vi "WritePointToMem.vi"(10 "Point":cluster{"X":i32, "Y":i32, "Z":i32}, 11 "PointNum":u32) -> ()   [LabVIEW 2014]
uses:
  <vilib>/Platform/TimedLoop/XDataNode/timing_clust.ctl
  <vilib>/Platform/TimedLoop/XDataNode/nitl_modes.ctl
  <vilib>/Platform/TimedLoop/XDataNode/wakeup.ctl
  <vilib>/rvi/Emulation/niFpgaSctlEmulationGetInTimedLoop.vi
  <vilib>/rvi/Emulation/niFpgaEmulationReportErrorSimple.vi
  <vilib>/rvi/Emulation/niFpgaGetClockAttributes.vi
  <vilib>/rvi/Emulation/niFpgaCriticalErrorInLSC.vi
  <vilib>/rvi/eio/common/nirviEmuTemplateMethod_errors.vi
  <vilib>/Platform/TimedLoop/XDataNode/XDataNode.xnode
  <vilib>/eio/EIONode/EIONode.xnode
  <vilib>/Platform/TimedLoop/XDataNode/XDNodeRunTimeDep.lvlib
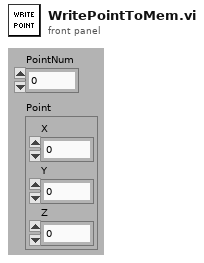
[diagram p1: front panel]
types:
  T1 = typedef "XDNodeRunTimeDep.lvlib/timing_clust.ctl" = cluster{"Expected End [f-1]":u64, "Actual End [f-1]":u64, "Finished Late? [f-1]":bool, "Expected End [i-1]":u64, "Actual End [i-1]":u64, "Finished Late? [i-1]":bool, "Expected Start [i]":u64, "Actual Start [i]":u64, "Expected Start [f]":u64, "Actual Start [f]":u64, "Source Name":string, "Structure Name":string, "Period":i64, "Deadline":i64, "Offset":i64, "Start":i64, "Priority":i32, "Timeout":i32, "Mode":T2, "Wakeup Reason":T3, "Error":errorcluster, "Source Type":string, "Secondary Source Type":string, "Global End Time":u64, "Global Start Time":u64, "Frame Duration":u64, "Iteration Duration":u64, "Assigned CPU":i32, "I/O Scan Engine Mode":u32}
  T2 = typedef "XDNodeRunTimeDep.lvlib/nitl_modes.ctl" = enum32{"No Change", "Process missed periods, maintain original phase", "Discard missed periods, maintain original phase", "Process missed periods, ignore original phase", "Discard missed periods, ignore original phase"}
  T3 = typedef "XDNodeRunTimeDep.lvlib/wakeup.ctl" = enum32{"Normal", "Aborted", "Asynchronous wakeup", "Timing source error", "Timed loop error", "Timeout"}
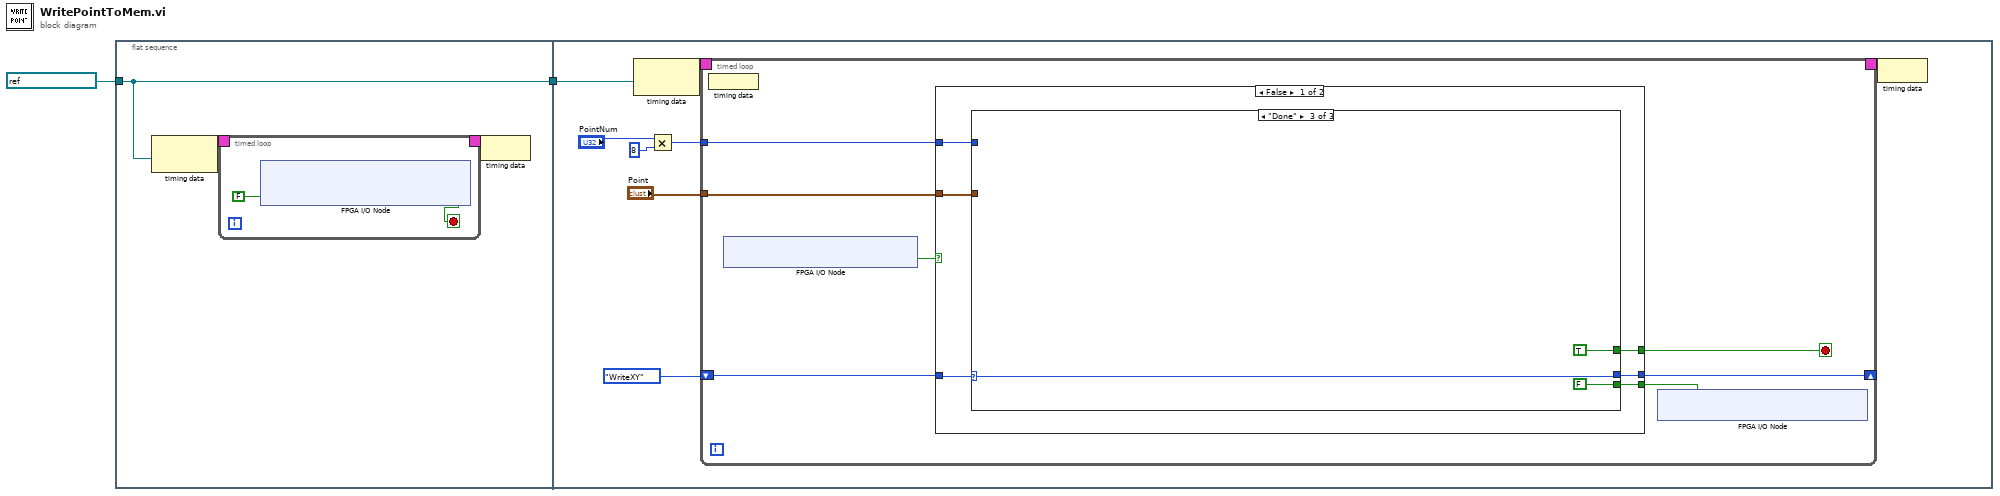
[diagram p0: block diagram]
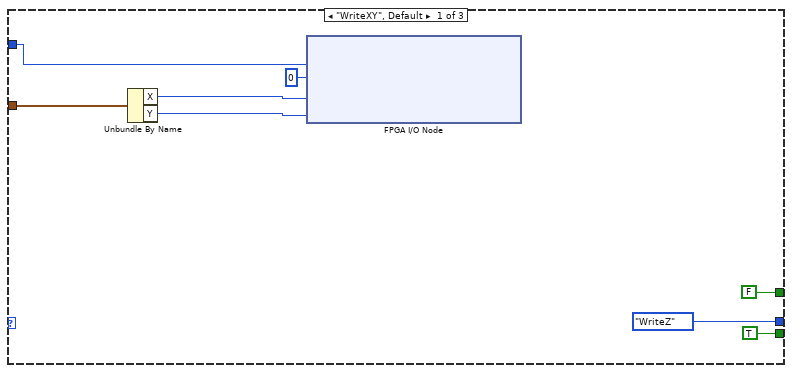
[diagram p2: hidden frame]
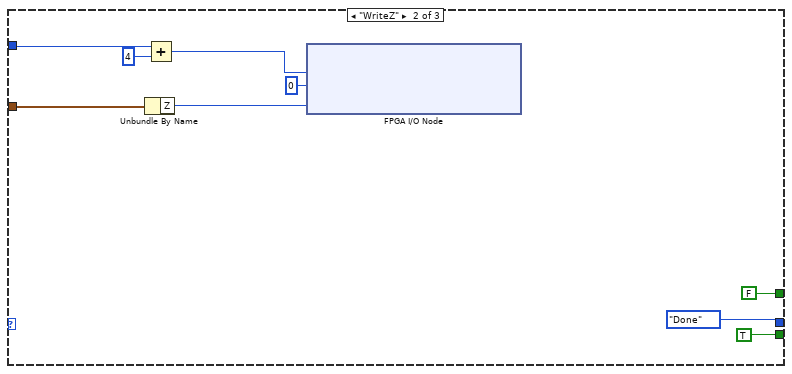
[diagram p3: hidden frame]
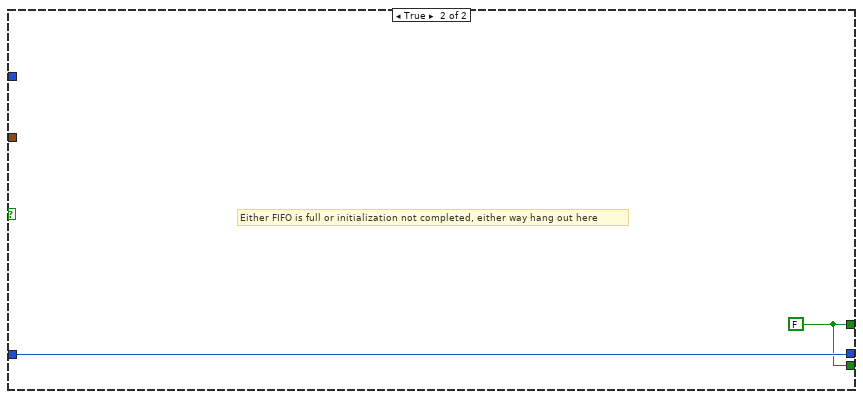
[diagram p4: hidden frame]
diagram:
  n1 = flat-sequence {
    tunnel: refnum<k21> "100 MHz Clock" ("Source Name") -> [w3]
    tunnel: [w3] -> w1
    tunnel: w1 -> [w14]
    frame #0 {
      n2 = node-c288(w3) -> (w5:T1)
      n3 = timed-loop {
        timing: w5 -> [_]
        timing-out: [_] -> w4
        stop <- w7 stop-if-true
        n4 = xnode "FPGA I/O Node"("DRAM Bank 0\\Command_Write_Enable"=FALSE ("DRAM Bank 0\\Command_Write_Enable")) -> ("DRAM Bank 0\\Initialization_Done"=w7:bool)  [unwired: 2 in, 2 out]
      }
      n5 = node-c288(w4) -> ()
    }
    frame #1 {
      n6 = node-c288(w14) -> (w21:T1)
      n7 = Multiply(x="PointNum", y=i16 8) -> (x*y=w17:u32)
      n8 = timed-loop {
        timing: w21 -> [_]
        timing-out: [_] -> w20
        tunnel: w17 -> [w26]
        shift-right: [w24] -> _
        shift-left: enum16{"WriteXY", "WriteZ", "Done"}."WriteXY" -> [w27]
        tunnel: "Point" -> [w25]
        stop <- w23 stop-if-true
        n9 = node-c288() -> ()  [unwired: 1 in]
        n10 = xnode "FPGA I/O Node"() -> ("DRAM Bank 0\\Command_FIFO_Full"=w22:bool)  [unwired: 1 in, 1 out]
        n11 = case shown="False" w22 {
          tunnel: [w34 w56] -> w28
          tunnel: w27 -> [w35 w57]
          tunnel: w26 -> [w33 _]
          tunnel: w25 -> [w32 _]
          tunnel: [w31 w57] -> w24
          tunnel: [w30 w56] -> w23
          frame False {
            n12 = case shown="\"Done\"" w35 {
              selector: w35 -> [_ _ w54]
              tunnel: [TRUE TRUE FALSE] -> w34
              tunnel: w33 -> [w43 w49 _]
              tunnel: w32 -> [w40 w46 _]
              tunnel: [enum16{"WriteXY", "WriteZ", "Done"}."WriteZ" enum16{"WriteXY", "WriteZ", "Done"}."Done" w54] -> w31
              tunnel: [FALSE FALSE TRUE] -> w30
              frame "WriteXY", Default {
                n13 = Unbundle By Name(w40) -> ("X"=w39:i32, "Y"=w38:i32)
                n14 = xnode "FPGA I/O Node"("DRAM Bank 0\\Address"=w43, "DRAM Bank 0\\Command"=u8 0 ("DRAM Bank 0\\Command"), "DRAM Bank 0\\Write_Data_Upper"=w39, "DRAM Bank 0\\Write_Data_Lower"=w38) -> ()  [unwired: 4 in, 4 out]
              }
              frame "WriteZ" {
                n15 = Unbundle By Name(w46) -> ("Z"=w45:i32)
                n16 = Add(x=w49, y=u32 4) -> (x+y=w47:u32)
                n17 = xnode "FPGA I/O Node"("DRAM Bank 0\\Address"=w47, "DRAM Bank 0\\Command"=u8 0 ("DRAM Bank 0\\Command"), "DRAM Bank 0\\Write_Data_Upper"=w45) -> ()  [unwired: 3 in, 3 out]
              }
              frame "Done" {
              }
            }
          }
          frame True {
            w56 = FALSE
            # "Either FIFO is full or initialization not completed, either way hang out here"
          }
        }
        n18 = xnode "FPGA I/O Node"("DRAM Bank 0\\Command_Write_Enable"=w28) -> ()  [unwired: 1 in, 1 out]
      }
      n19 = node-c288(w20) -> ()
    }
  }
